vi "System_Read Asset Objects.vi"(11 "data value reference":refnum<data-value>) -> (2 "Asset DVR Array":refnum<data-value>[](array[refnum]), 3 "data value reference out":refnum<data-value>)   [LabVIEW 2015, in "System.lvclass"]
uses:
  System.lvclass
  AssetInterface.lvclass
  System.lvclass/System.ctl
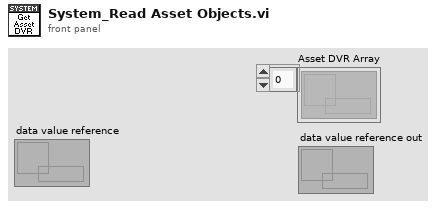
[diagram p1: front panel]
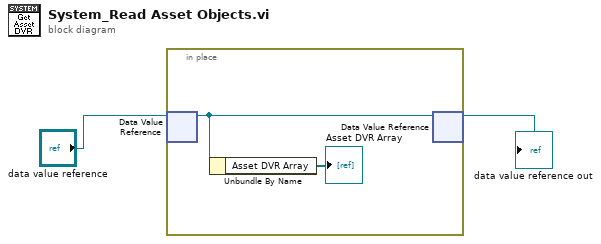
[diagram p0: block diagram]
diagram:
  n1 = in-place {
    n2 = in-place-dvr #1("data value reference") -> (w4:refnum<class "System.lvclass">)  [unwired: 1 out]
    n3 = Unbundle By Name(w4) -> ("Asset DVR Array"=→"Asset DVR Array":refnum<data-value>[])
    n4 = in-place-dvr #1(w4) -> (→"data value reference out":refnum<data-value>)  [unwired: 1 out]
  }
